vi "Send-Receive Serial Port.vi"(0 "Data to write":string, 11 "error in (no error)":errorcluster) -> (4 "Data read":string, 15 "error out":errorcluster)   [LabVIEW 2024, in "GRBL 1.1.lvlib"]
doc: "This VI send and receive data on serial port of the selected controller."
uses:
  GRBL 1.1.lvlib
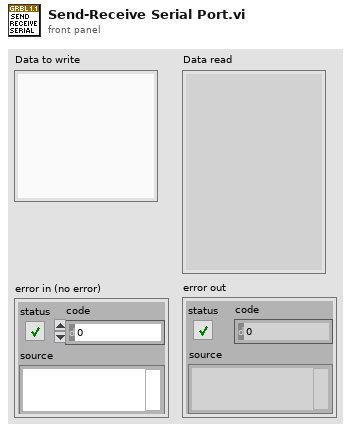
[diagram p1: front panel]
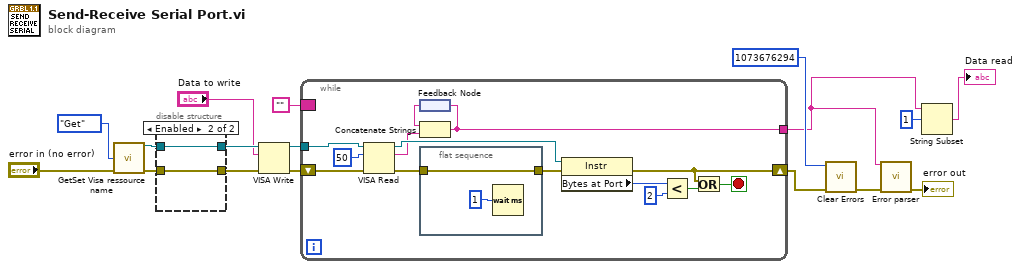
[diagram p0: block diagram]
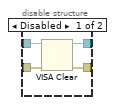
[diagram p2: hidden frame]
diagram:
  n1 = call "GetSet Visa ressource name.vi"("Get/Set"=enum16{"Get", "Set"}."Get", "error in (no error)"="error in (no error)") -> ("VISA resource name out"=w10:refnum<visa-resource-name>, "error out"=w12:errorcluster)  [unwired: 12 in]
  n2 = disable-structure shown="Enabled" {
    disable-tunnel: w12 -> [w21 w22]
    disable-tunnel: [w20 w23] -> w11
    disable-tunnel: w10 -> [w19 w23]
    disable-tunnel: [w18 w22] -> w8
    frame Disabled {
      n3 = VISA Clear(VISA resource name=w19, error in (no error)=w21) -> (VISA resource name out=w20:refnum<visa-resource-name>, error out=w18:errorcluster)
    }
    frame Enabled {
    }
  }
  n4 = VISA Write(VISA resource name=w11, write buffer="Data to write", error in (no error)=w8) -> (VISA resource name out=w7:refnum<visa-resource-name>, error out=w6:errorcluster)  [unwired: 1 out]
  n5 = while {
    tunnel: w7 -> [w37]
    tunnel: [w32] -> w3
    shift-right: [w28] -> w1
    shift-left: w6 -> [w36]
    border: "" -> [_]
    stop <- w29 stop-if-true
    n6 = VISA Read(VISA resource name=w37, byte count=u32 50, error in (no error)=w36) -> (VISA resource name out=w34:refnum<visa-resource-name>, read buffer=w27:string, error out=w26:errorcluster)  [unwired: 1 out]
    n7 = feedback #1() -> (w33:string)
    n8 = Concatenate Strings(w33, w27) -> (w32:string)
    n9 = feedback-in #1(w32) -> ()
    n10 = flat-sequence {
      tunnel: w26 -> [w38]
      tunnel: [w38] -> w25
      frame #0 {
        n11 = Wait (ms)(milliseconds to wait=u32 1) -> ()  [unwired: 1 out]
      }
    }
    n12 = property class="Instr"(reference=w34, error in=w25) -> (error out=w28:errorcluster, "Bytes at Port"=w24:u32)  [unwired: 1 out]
    n13 = Less?(x=w24, y=u32 2) -> (x < y?=w31:bool)
    n14 = Or(x=w28, y=w31) -> (x .or. y?=w29:bool)
  }
  n15 = call <vilib>:"Clear Errors.vi"("error in (no error)"=w1, "specific error code to clear (0: all)"=1073676294 ("error code (0)")) -> ("error out"=w13:errorcluster)  [unwired: 4 in, 1 out]
  n16 = call "Error parser.vi"("Data Readed"=w3, "error in (no error)"=w13) -> ("error out"=→"error out":errorcluster)  [unwired: 13 in]
  n17 = String Subset(string=w3, offset (0)=1) -> (substring=→"Data read":string)  [unwired: 1 in]
